vi "Import Parameters Configuration to New AIM ARINC 664 Custom Device.vi"(6 "Bin File Parameter Data":path=path "Support/2FrameProperlyDefined.bin", 7 "Base System Definition File":path=path "Support/Base.nivssdf", 9 "Parameters Configuration File":path=path "Support/UDP_RX_TX_Loopback_TxRxMon.xml", 11 "Output System Definition File":path=path "Support/Imported AIM ARINC 664.nivssdf") -> (3 "AIM ARINC 664 System Definition":path)   [LabVIEW 2020]
doc: "Overview: Demonstrates using the AIM ARINC 664 scripting API to configure the custom device by importing a parameters configuration file. \n\nInstructions:\n1. Specify the Parameters Configuration File. This parameters configuration file must be consistent with the schema published on the GitHub repo (https://github.com/ni/niveristand-aim-arinc664-custom-device/blob/main/Docs/Parameters%20XML%20File/ARINC664_Parameters_XML_Schema.xsd). For successful deployment, the parameters configuration file must also be consistent with the hardware configuration file.\n2. Specify the Hardware Configuration File. The hardware configuration file must be consistent with the schema installed by the Ballard hardware driver at C:\\Program Files (x86)\\Astronics Ballard Technology LabVIEW Driver\\Help\\index.html.\n3. (VeriStand) Optionally, you may open the AIM ARINC 664 System Definition in VeriStand, configure the PXI Linux RT Target, and deploy the scripted system definition to perform avionics bus communications with AIM ARINC 664 hardware."
uses:
  AIM ARINC 664 Scripting Examples.lvlib
  <vilib>/addons/VeriStand Custom Device Scripting APIs/AIM ARINC 664/Scripting/AIM ARINC 664 Scripting.lvlib
  NationalInstruments.VeriStand.SystemDefinitionAPI
panel:
  # "Overview: Demonstrates using the AIM ARINC 664 scripting API to configure the custom device by importing a parameters configuration file. \n\nInstructions:\n1. Specify the Parameters Configuration File. This parameters configuration file must be consistent with the schema published on the GitHub repo (https://github.com/ni/niveristand-aim-arinc664-custom-device/blob/main/Docs/Parameters%20XML%20File/ARINC664_Parameters_XML_Schema.xsd).\n3. (VeriStand) Optionally, you may open the AIM ARINC 664 System Definition in VeriStand, configure the PXI Linux RT Target, and deploy the scripted system definition to perform avionics bus communications with AIM ARINC 664 hardware."
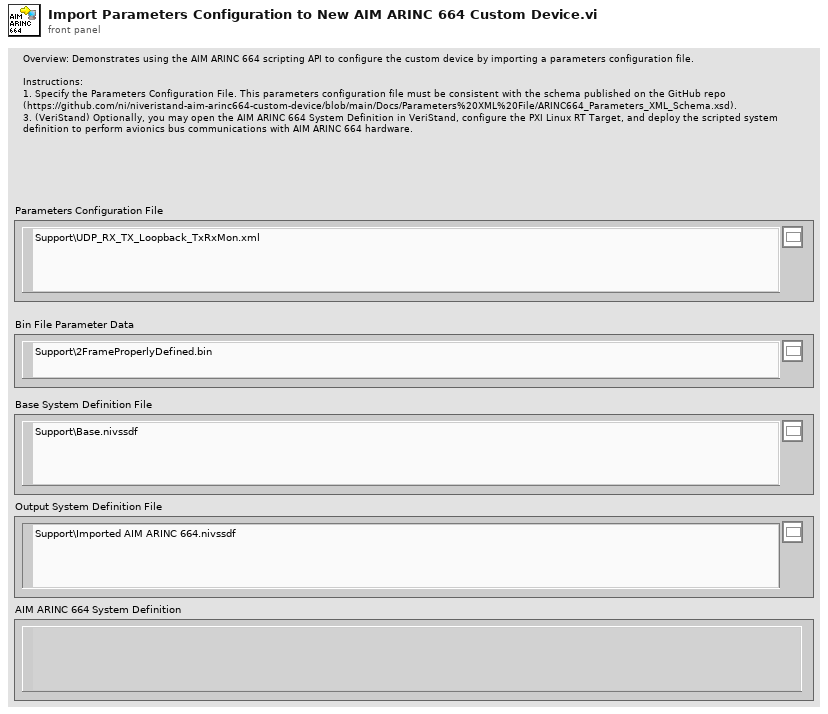
[diagram p1: front panel]
types:
  T1 = typedef "Custom Device API.lvlib/Custom Device Item Ref.ctl" = u64
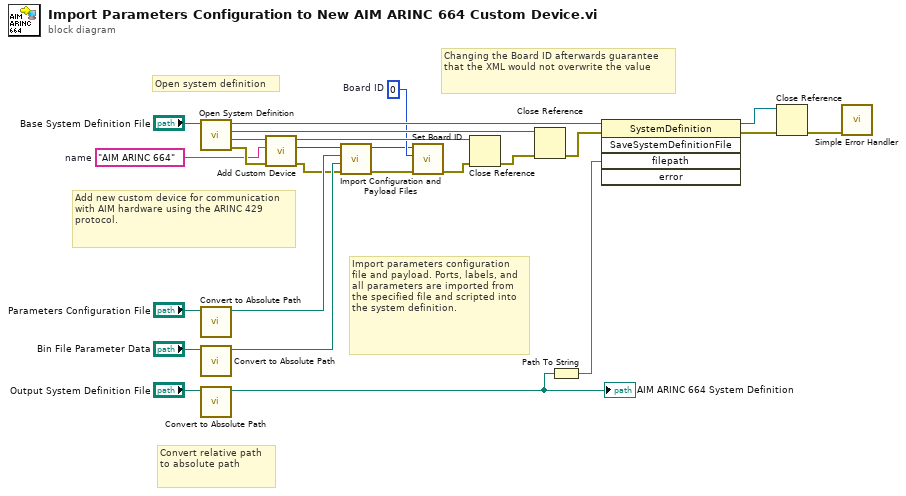
[diagram p0: block diagram]
diagram:
  w8 = 0  # Board ID
  w13 = "AIM ARINC 664"  # name
  # "Changing the Board ID afterwards guarantee that the XML would not overwrite the value"
  # "Import parameters configuration file and payload. Ports, labels, and all parameters are imported from the specified file and scripted into the system definition."
  # "Add new custom device for communication with AIM hardware using the ARINC 429 protocol."
  # "Convert relative path to absolute path"
  # "Open system definition"
  # "8."
  n1 = call "Open System Definition.vi"("system definition file"="Base System Definition File") -> ("error out"=w14:errorcluster, "target"=w15:refnum<k24>, "root"=w17:refnum<k24>, "system definition"=w18:refnum<k24>)  [unwired: 7 in]
  n2 = call "Convert to Absolute Path.vi"("system definition file"="Parameters Configuration File") -> ("absolute path"=w11:path)  [unwired: 10 in]
  n3 = call "Convert to Absolute Path.vi"("system definition file"="Bin File Parameter Data") -> ("absolute path"=w6:path)  [unwired: 10 in]
  n4 = call "Convert to Absolute Path.vi"("system definition file"="Output System Definition File") -> ("absolute path"=w9:path)  [unwired: 10 in]
  "AIM ARINC 664 System Definition" <- w9
  n5 = call <vilib>:"Add Custom Device.vi"("error in"=w14, "name"=w13, "target in"=w15) -> ("error out"=w3:errorcluster, "custom device"=w5:T1, "target out"=w10:refnum<k24>)  [unwired: 6 in]
  n6 = call <vilib>:"Import Configuration and Payload Files.vi"("error in"=w3, "payload file path"=w6, "parameters configuration file path"=w11, "custom device ref"=w5) -> ("error out"=w2:errorcluster, "custom device ref out"=w4:T1)  [unwired: 6 in]
  n7 = call <vilib>:"Set Board ID.vi"("error in"=w2, "Board ID"=w8, "custom device ref"=w4) -> ("error out"=w1:errorcluster)  [unwired: 7 in, 1 out]
  n8 = Close Reference(reference=w10, error in (no error)=w1) -> (error out=w16:errorcluster)
  n9 = Close Reference(reference=w17, error in (no error)=w16) -> (error out=w21:errorcluster)
  n10 = Path To String(path=w9) -> (string=w24:string)
  n11 = invoke class="SystemDefinition" method="SaveSystemDefinitionFile"(reference=w18, error in=w21, "filepath"=w24) -> (reference out=w22:refnum<k24>, error out=w23:errorcluster)  [unwired: 2 in, 3 out]
  n12 = Close Reference(reference=w22, error in (no error)=w23) -> (error out=w20:errorcluster)
  n13 = call <vilib>:"Simple Error Handler.vi"("error in (no error)"=w20) -> ()  [unwired: 1 in, 8 out]
